vi "Step 5 - Generate Decimation for FPGA (MRate).vi"() -> ()   [LabVIEW 2023]
doc: "Demonstrates how to use the DFD FXP MRate Code Generator VI to generate LabVIEW field-programmable gate array (FPGA) code.\n\nComplete the following steps to use this VI.\n1) Set the <B>Destination Folder</B> that contains all the generated VIs and the LabVIEW project.\n2) Run the VI.\n3) The <B>Max Input Fs@40 MHz FPGA Clock</B> returns a value that indicates the processing power of the generated filter block.\n\nWhen this VI finishes generating the LabVIEW FPGA code, this VI opens the generated LabVIEW project automatically."
uses:
  <vilib>/addons/Digital Filter Design/_Objects.llb/DFD Coef Norm Type.ctl
  <vilib>/addons/Digital Filter Design/NI_DigFilterLicensed.lvlib
panel:
  in  "# Channels":i32=1
  out "Maximum Input Fs@40 MHz FPGA Clock":dbl format="%#_5p Hz"
  in  "Filter Name":string="MRate_Decimation"
  in  "Destination Folder":path
  # "Select Help>>Show Context Help and move the cursor over the VI icon for more information."
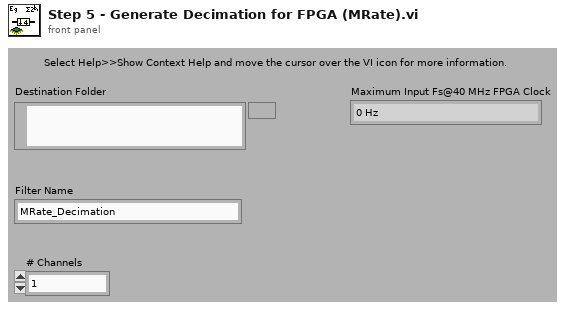
[diagram p1: front panel]
types:
  T1 = typedef "NI_DigFilterLicensed.lvlib/DFD Coef Norm Type.ctl" = enum16{"No Norm", "Time Domain 1-Norm", "Time Domain 2-Norm", "Time Domain Inf-Norm"}
  T2 = typedef "NI_DigFilterLicensed.lvlib/DFD Multirate Filter Obj.ctl" = cluster{"mMRate_Structure":enum16{"CIC", "FIR", "IIR", "Lattice"}, "mMRate_Mode":T3, "mMRate_Factor":i32, "mMRate_FIRParams":cluster{"mMRate_FIR_H":dbl[], "mMRate_FIR_IsNyquist?":bool, "mMRate_FIR_IsSymmetric?":bool}, "mMRate_CICParams":cluster{"mMRate_CIC_#Stage":i32, "mMRate_CIC_Lag":i32, "mMRate_CIC_Type":enum16{"Lowpass", "Highpass"}}, "mMRate_Order":i32, "mMRate_Version":string, "mMRate_Comments":string, "mMRate_RationalFactor":cluster{"mMRate_L":i32, "mMRate_M":i32}, "mMRate_Fs":dbl, "mMRate_Quantized?":bool, "mMRate_QFilterGain":dbl, "mMRate_CoefWl":i16, "mMRate_Scaling":cluster{"mMRate_ScaleByPowerOf2?":bool, "mMRate_ScaleType":T1}, "mMRate_InputWl":i16, "mMRate_OutputWl":i16, "mMRate_OutputMode":T4, "mMRate_MultMode":T5, "mMRate_BitPruning":bool, "mMRate_GainWl":i16, "mMRate_OutputFwl":i16, "mMRate_SumIwl":i16, "mMRate_InputIwl ":i16, "mMRate_SumWl":i16, "mMRate_CoefIwl":i16}
  T3 = typedef "NI_DigFilterLicensed.lvlib/DFD Multirate Mode.ctl" = i16
  T4 = typedef "NI_DigFilterLicensed.lvlib/DFD Round-off Mode.ctl" = enum16{"Nearest", "Truncation"}
  T5 = typedef "NI_DigFilterLicensed.lvlib/DFD FXP MRate Multiply Mode.ctl" = enum16{"Truncated", "Full"}
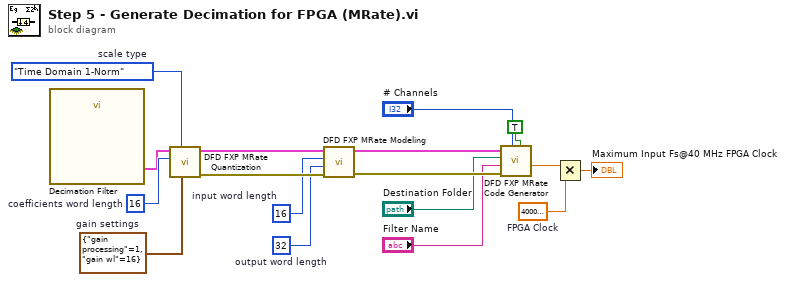
[diagram p0: block diagram]
diagram:
  w3 = i16 16  # coefficients word length
  w4 = i16 32  # output word length
  w5 = i16 16  # input word length
  w6 = 40000000.0  # FPGA Clock
  w2 = cluster{"gain processing":u16, "gain wl":i16} {"gain processing"=1, "gain wl"=16}  # gain settings
  w17 = DFD_Coef_Norm_Type."Time Domain 1-Norm"  # scale type
  n1 = call "Decimation Filter"() -> ("multirate filter out"=w1:T2)  [unwired: 11 out]
  n2 = call <vilib>:"DFD FXP MRate Quantization.vi"("gain settings"=w2, "scale type"=w17, "coefficients word length"=w3, "multirate filter in"=w1) -> ("error out"=w15:errorcluster, "multirate filter out"=w16:T2)  [unwired: 2 in, 4 out]
  n3 = call <vilib>:"DFD FXP MRate Modeling.vi"("error in (no error)"=w15, "output word length"=w4, "input word length"=w5, "multirate filter in"=w16) -> ("error out"=w13:errorcluster, "multirate filter out"=w14:T2)  [unwired: 4 in, 2 out]
  n4 = call <vilib>:"DFD FXP MRate Code Generator.vi"("open project? (F)"=TRUE, "# channels"="# Channels", "error in (no error)"=w13, "filter name"="Filter Name", "destination folder"="Destination Folder", "multirate filter"=w14) -> ("sampling frequency/FPGA clock"=w9:dbl)  [unwired: 1 in, 4 out]
  n5 = Multiply(x=w9, y=w6) -> (x*y=→"Maximum Input Fs@40 MHz FPGA Clock":dbl)
